vi "ActiveX对excel操作范例.vi"() -> ()   [LabVIEW 2014]
panel:
  in  "字符串":string
  out "元素":i32
  in  "数组":string[][](array[string])
  out "错误输出":errorcluster
  out "数据":string[][](array[string])
  in  "excel路径":path
  in  "excel是否可见":bool
  in  "错误输入（无错误）":errorcluster
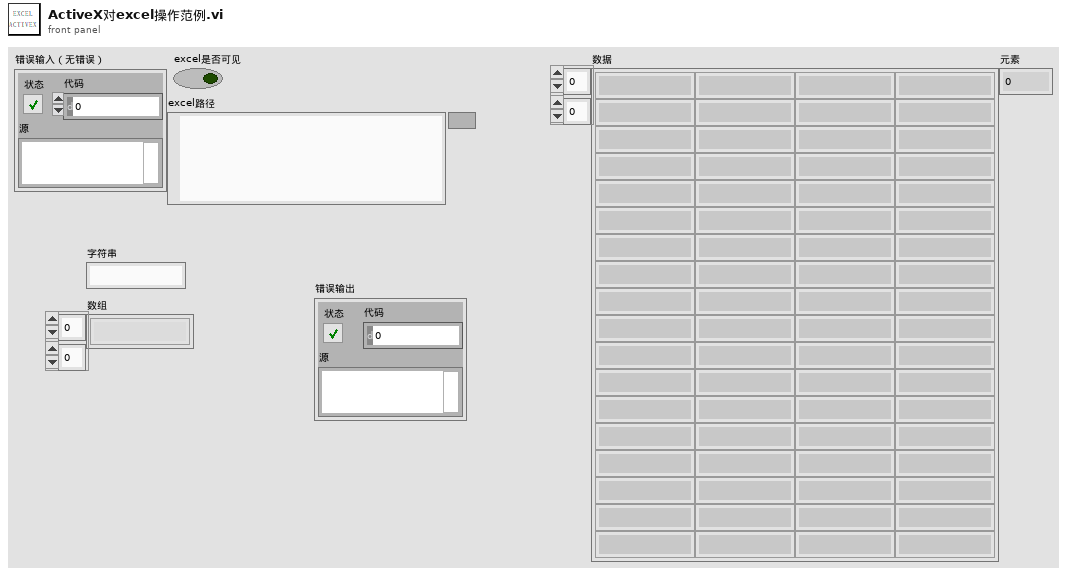
[diagram p1: front panel]
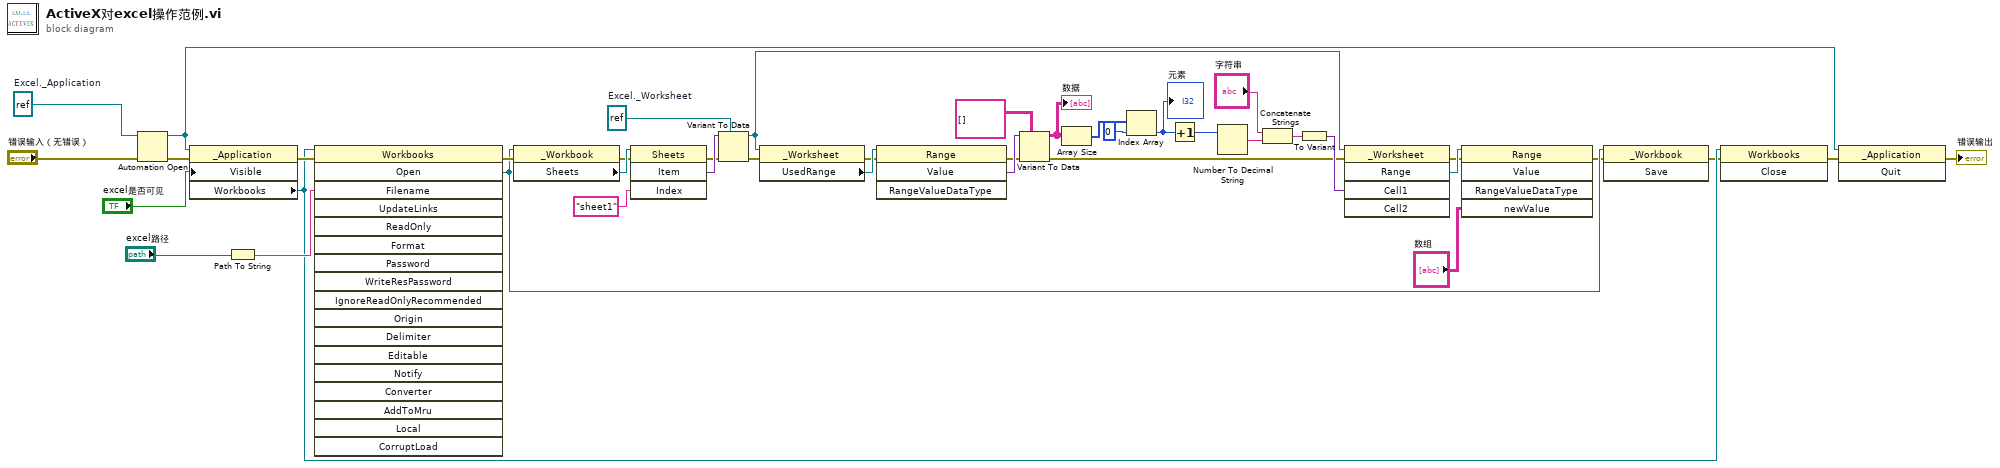
[diagram p0: block diagram]
diagram:
  w32 = refnum<k7> refnum  # Excel._Worksheet
  w41 = refnum<k7> refnum  # Excel._Application
  n1 = Automation Open(error in (no error)="错误输入（无错误）", Automation Refnum=w41) -> (Automation Refnum=w21:refnum<k7>, error out=w19:errorcluster)  [unwired: 2 in]
  n2 = property class="_Application"(reference=w21, error in=w19, "Visible"="excel是否可见") -> (error out=w38:errorcluster, "Workbooks"=w22:refnum<k7>)  [unwired: 1 out]
  n3 = Path To String(path="excel路径") -> (string=w37:string)
  n4 = invoke class="Workbooks" method="Open"(reference=w22, error in=w38, "Filename"=w37) -> (error out=w23:errorcluster, "Open"=w3:refnum<k7>)  [unwired: 15 in, 16 out]
  n5 = property class="_Workbook"(reference=w3, error in=w23) -> (error out=w30:errorcluster, "Sheets"=w35:refnum<k7>)  [unwired: 1 out]
  n6 = invoke class="Sheets" method="Item"(reference=w35, error in=w30, "Index"="sheet1" ("字符串")) -> (error out=w31:errorcluster, "Item"=w33:variant)  [unwired: 1 in, 2 out]
  n7 = Variant To Data(error in=w31, type=w32, Variant=w33) -> (data=w12:refnum<k7>, error out=w29:errorcluster)
  n8 = property class="_Worksheet"(reference=w12, error in=w29) -> (error out=w27:errorcluster, "UsedRange"=w28:refnum<k7>)  [unwired: 1 out]
  n9 = invoke class="Range" method="Value"(reference=w28, error in=w27) -> (error out=w25:errorcluster, "Value"=w26:variant)  [unwired: 2 in, 2 out]
  n10 = Variant To Data(error in=w25, type=string[][] [] ("数组"), Variant=w26) -> (data=w17:string[][], error out=w9:errorcluster)
  "数据" <- w17
  n11 = Array Size(array=w17) -> (size(s)=w16:i32[])
  n12 = Index Array(array=w16, index=0 ("索引")) -> (element=w6:i32)
  "元素" <- w6
  n13 = Increment(x=w6) -> (x+1=w5:i32)
  n14 = Number To Decimal String(number=w5) -> (decimal integer string=w4:string)  [unwired: 1 in]
  n15 = Concatenate Strings("字符串", w4) -> (w8:string)
  n16 = To Variant(anything=w8) -> (Variant=w11:variant)
  n17 = invoke class="_Worksheet" method="Range"(reference=w12, error in=w9, "Cell1"=w11) -> (error out=w13:errorcluster, "Range"=w14:refnum<k7>)  [unwired: 2 in, 3 out]
  n18 = invoke class="Range" method="Value"(reference=w14, error in=w13, "newValue"="数组") -> (error out=w2:errorcluster)  [unwired: 2 in, 4 out]
  n19 = invoke class="_Workbook" method="Save"(reference=w3, error in=w2) -> (error out=w1:errorcluster)  [unwired: 1 in, 2 out]
  n20 = invoke class="Workbooks" method="Close"(reference=w22, error in=w1) -> (error out=w20:errorcluster)  [unwired: 1 in, 2 out]
  n21 = invoke class="_Application" method="Quit"(reference=w21, error in=w20) -> (error out=→"错误输出":errorcluster)  [unwired: 1 in, 2 out]
